vi "Edge-Quad intersection test.vi"(2 "Quad":T1, 3 "Edge vector (not unit)":sgl[](array[numeric]), 4 "Edge start point":sgl[](array[numeric])) -> (0 "Intersection point":sgl[](array[numeric]), 1 "Intersection":bool)   [LabVIEW 2014]
uses:
  Typedefs/Quad.ctl
panel:
  # "PN 17/01/2015"
  # "Vertices"
  # "Edges"
  # "Unit normal"
  # "Edge unit normals"
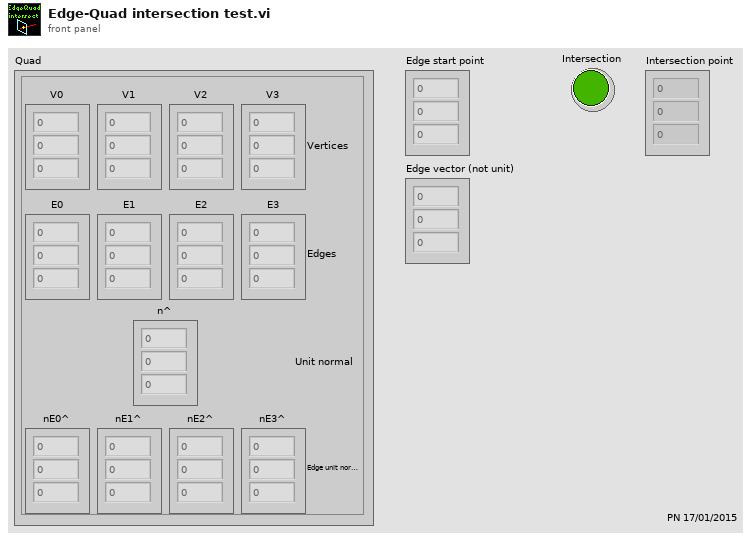
[diagram p1: front panel]
types:
  T1 = typedef "Quad.ctl" = cluster{"V0":sgl[], "V1":sgl[], "V2":sgl[], "V3":sgl[], "E0":sgl[], "E1":sgl[], "E2":sgl[], "E3":sgl[], "n^":sgl[], "nE0^":sgl[], "nE1^":sgl[], "nE2^":sgl[], "nE3^":sgl[]}
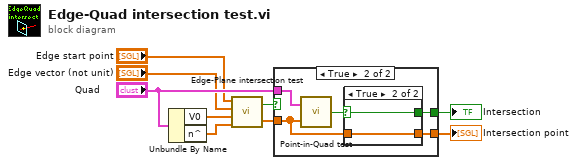
[diagram p0: block diagram]
diagram:
  n1 = Unbundle By Name("Quad") -> ("V0"=w7:sgl[], "n^"=w8:sgl[])
  n2 = call "Edge-Plane intersection test.vi"("Plane normal (unit)"=w8, "Point on plane"=w7, "Edge vector (not unit)"="Edge vector (not unit)", "Edge start point"="Edge start point") -> ("Intersection point"=w6:sgl[], "Intersection"=w5:bool)
  n3 = case shown="True" w5 {
    selector: w5 -> [w10 _]
    tunnel: w6 -> [_ w13]
    tunnel: "Quad" -> [_ w15]
    tunnel: [w10 w12] -> w2
    tunnel: [_ w11] -> w1
    frame False {
    }
    frame True {
      n4 = call "Point-in-Quad test.vi"("Point"=w13, "Quad"=w15) -> ("Point is inside quad"=w14:bool)
      n5 = case shown="True" w14 {
        selector: w14 -> [w16 w18]
        tunnel: w13 -> [_ w17]
        tunnel: [w16 w18] -> w12
        tunnel: [_ w17] -> w11
        frame False {
        }
        frame True {
        }
      }
    }
  }
  "Intersection" <- w2
  "Intersection point" <- w1
